vi "InternalResistance.vi"   [LabVIEW 2015]
uses:
  Formula Hybrid 2012 r1/Global Data.vi
  <vilib>/Platform/TimedLoop/XDataNode/XDataNode.xnode
  <vilib>/Platform/TimedLoop/XDataNode/nitl_modes.ctl
  <vilib>/Platform/TimedLoop/XDataNode/XDNodeRunTimeDep.lvlib
  <vilib>/Platform/TimedLoop/XDataNode/wakeup.ctl
  <vilib>/Platform/TimedLoop/XDataNode/timing_clust.ctl
types:
  T1 = typedef "XDNodeRunTimeDep.lvlib/timing_clust.ctl" = cluster{"Expected End [f-1]":u64, "Actual End [f-1]":u64, "Finished Late? [f-1]":bool, "Expected End [i-1]":u64, "Actual End [i-1]":u64, "Finished Late? [i-1]":bool, "Expected Start [i]":u64, "Actual Start [i]":u64, "Expected Start [f]":u64, "Actual Start [f]":u64, "Source Name":string, "Structure Name":string, "Period":i64, "Deadline":i64, "Offset":i64, "Start":i64, "Priority":i32, "Timeout":i32, "Mode":T2, "Wakeup Reason":T3, "Error":errorcluster, "Source Type":string, "Secondary Source Type":string, "Global End Time":u64, "Global Start Time":u64, "Frame Duration":u64, "Iteration Duration":u64, "Assigned CPU":i32, "I/O Scan Engine Mode":u32}
  T2 = typedef "XDNodeRunTimeDep.lvlib/nitl_modes.ctl" = enum32{"No Change", "Process missed periods, maintain original phase", "Discard missed periods, maintain original phase", "Process missed periods, ignore original phase", "Discard missed periods, ignore original phase"}
  T3 = typedef "XDNodeRunTimeDep.lvlib/wakeup.ctl" = enum32{"Normal", "Aborted", "Asynchronous wakeup", "Timing source error", "Timed loop error", "Timeout"}
  T4 = typedef "BMS Telemetry.ctl" = cluster{"bBMSIgnition":bool, "bBMSChargerMains":bool, "bBMSFastCharge":bool, "bBMSChargerEnabled":bool, "eBMSCarState":enum16{"Off", "On, Not Charging", "Charging", "Charging Finished", "Charging Error"}, "eBMSChargingState":enum16{"Disconnected", "Pre-charging", "Main Charging", "Balancing", "Charging Finished OK", "Charging Error"}, "tBMSChargeStage":u16, "eBMSLastChargeError":enum16{"No Error", "No Cell Communication", "No Cell Communication - Non CAN Charger", "Maximum charging stage duration expired", "Cell Communication Lost during Charge", "Cannot set balancing voltage", "Cell temps too high", "No Comms so can't determine temp", "# of Cells Mismatch", "Cells Overvoltage", "Cell Protection Event occured."}, "NBMSNumCells":u8, "bBMSUnderVProtection":bool, "bBMSOverVProtection":bool, "bBMSOverTProtection":bool, "bBMSLeakageProtection":bool, "bBMSNoCellCommsError":bool, "bBMSLowVReduction":bool, "bBMSHighTReduction":bool, "VCellMin":dbl, "VCellMax":dbl, "VCellMean":dbl, "VTotal":dbl, "TCellMin":dbl, "TCellMax":dbl, "TCellMean":dbl, "VCells":cluster{"[0]":dbl, "[1]":dbl, "[2]":dbl, "[3]":dbl, "[4]":dbl, "[5]":dbl, "[6]":dbl, "[7]":dbl, "[8]":dbl, "[9]":dbl, "[10]":dbl, "[11]":dbl, "[12]":dbl, "[13]":dbl, "[14]":dbl, "[15]":dbl, "[16]":dbl, "[16] 2":dbl, "[17]":dbl, "[18]":dbl, "[19]":dbl, "[20]":dbl, "[21]":dbl, "[22]":dbl, "[23]":dbl, "[24]":dbl, "[25]":dbl, "[26]":dbl, "[27]":dbl, "[28]":dbl, "[29]":dbl, "[30]":dbl, "[31]":dbl, "[32]":dbl, "[33]":dbl, "[33] 2":dbl, "[34]":dbl, "[35]":dbl, "[36]":dbl, "[37]":dbl, "[38]":dbl, "[39]":dbl, "[40]":dbl, "[41]":dbl, "[42]":dbl, "[43]":dbl, "[44]":dbl, "[45]":dbl, "[46]":dbl, "[47]":dbl, "[48]":dbl, "[49]":dbl, "[50]":dbl, "[50] 2":dbl, "[51]":dbl, "[52] 2":dbl, "[54]":dbl, "[53]":dbl, "[55]":dbl, "[56]":dbl, "[57]":dbl, "[58]":dbl, "[59]":dbl, "[60]":dbl, "[61]":dbl, "[62]":dbl, "[63]":dbl, "[64]":dbl, "[65]":dbl, "[66]":dbl, "[67]":dbl}, "TBMSCells":cluster{"[55]":dbl, "[56]":dbl, "[57]":dbl, "[58]":dbl, "[59]":dbl, "[60]":dbl, "[61]":dbl, "[62]":dbl, "[63]":dbl, "[64]":dbl, "[65]":dbl, "[66]":dbl, "[67]":dbl, "[68]":dbl, "[69]":dbl, "[70]":dbl, "[17]":dbl, "[38]":dbl, "[39]":dbl, "[40]":dbl, "[41]":dbl, "[42]":dbl, "[43]":dbl, "[44]":dbl, "[45]":dbl, "[46]":dbl, "[47]":dbl, "[48]":dbl, "[49]":dbl, "[50]":dbl, "[51]":dbl, "[52]":dbl, "[53]":dbl, "[54]":dbl, "[21]":dbl, "[22]":dbl, "[23]":dbl, "[24]":dbl, "[25]":dbl, "[26]":dbl, "[27]":dbl, "[28]":dbl, "[29]":dbl, "[30]":dbl, "[31]":dbl, "[32]":dbl, "[33]":dbl, "[34]":dbl, "[35]":dbl, "[36]":dbl, "[37]":dbl, "[0]":dbl, "[1]":dbl, "[2]":dbl, "[3]":dbl, "[4]":dbl, "[5]":dbl, "[6]":dbl, "[7]":dbl, "[8]":dbl, "[9]":dbl, "[10]":dbl, "[11]":dbl, "[12]":dbl, "[13]":dbl, "[14]":dbl, "[15]":dbl, "[16]":dbl}, "bChargerConnected":bool, "VChargerSetpoint":dbl, "IChargerSetpoint":dbl, "VChargerActual":dbl, "IChargerActual":dbl, "BCells":cluster{"[51]":dbl, "[52]":dbl, "[53]":dbl, "[54]":dbl, "[55]":dbl, "[56]":dbl, "[57]":dbl, "[58]":dbl, "[59]":dbl, "[60]":dbl, "[61]":dbl, "[62]":dbl, "[63]":dbl, "[64]":dbl, "[65]":dbl, "[66]":dbl, "[67]":dbl, "[34]":dbl, "[35]":dbl, "[36]":dbl, "[37]":dbl, "[38]":dbl, "[39]":dbl, "[40]":dbl, "[41]":dbl, "[42]":dbl, "[43]":dbl, "[44]":dbl, "[45]":dbl, "[46]":dbl, "[47]":dbl, "[48]":dbl, "[49]":dbl, "[50]":dbl, "[17]":dbl, "[18]":dbl, "[19]":dbl, "[20]":dbl, "[21]":dbl, "[22]":dbl, "[23]":dbl, "[24]":dbl, "[25]":dbl, "[26]":dbl, "[27]":dbl, "[28]":dbl, "[29]":dbl, "[30]":dbl, "[31]":dbl, "[32]":dbl, "[33]":dbl, "[0]":dbl, "[1]":dbl, "[2]":dbl, "[3]":dbl, "[4]":dbl, "[5]":dbl, "[6]":dbl, "[7]":dbl, "[8]":dbl, "[9]":dbl, "[10]":dbl, "[11]":dbl, "[12]":dbl, "[13]":dbl, "[14]":dbl, "[15]":dbl, "[16]":dbl}, "bNewVCellMinSample":bool, "Battery Temp":cluster{"[0]":dbl, "[1]":dbl, "[2]":dbl, "[3]":dbl, "[4]":dbl, "[5]":dbl, "[6]":dbl, "[7]":dbl, "[8]":dbl, "[9]":dbl, "[10]":dbl, "[11]":dbl, "[12]":dbl, "[13]":dbl, "[14]":dbl, "[15]":dbl, "[16]":dbl, "[17]":dbl, "[18]":dbl, "[19]":dbl, "[20]":dbl, "[21]":dbl, "[22]":dbl, "[23]":dbl, "[24]":dbl, "[25]":dbl, "[26]":dbl, "[27]":dbl, "[28]":dbl, "[29]":dbl, "[30]":dbl, "[31]":dbl, "[32]":dbl, "[33]":dbl, "[34]":dbl, "[35]":dbl, "[36]":dbl, "[37]":dbl, "[38]":dbl, "[39]":dbl, "[40]":dbl, "[41]":dbl, "[42]":dbl, "[43]":dbl, "[44]":dbl, "[45]":dbl, "[46]":dbl, "[47]":dbl, "[48]":dbl, "[49]":dbl, "[50]":dbl, "[51]":dbl, "[52]":dbl, "[53]":dbl, "[54]":dbl, "[55]":dbl, "[56]":dbl, "[57]":dbl, "[58]":dbl, "[59]":dbl, "[60]":dbl, "[61]":dbl, "[62]":dbl, "[63]":dbl, "[64]":dbl, "[65]":dbl, "[66]":dbl, "[67]":dbl, "[68]":dbl, "[69]":dbl, "[70]":dbl, "[71]":dbl, "[0] 2":dbl, "[1] 2":dbl, "[2] 2":dbl, "[3] 2":dbl, "[4] 2":dbl, "[5] 2":dbl, "[6] 2":dbl, "[7] 2":dbl, "[8] 2":dbl, "[9] 2":dbl, "[10] 2":dbl, "[11] 2":dbl, "[12] 2":dbl, "[13] 2":dbl, "[14] 2":dbl, "[15] 2":dbl, "[16] 2":dbl, "[17] 2":dbl, "[18] 2":dbl, "[19] 2":dbl, "[20] 2":dbl, "[21] 2":dbl, "[22] 2":dbl, "[23] 2":dbl, "[24] 2":dbl, "[25] 2":dbl, "[26] 2":dbl, "[27] 2":dbl, "[28] 2":dbl, "[29] 2":dbl, "[30] 2":dbl, "[31] 2":dbl, "[32] 2":dbl, "[33] 2":dbl, "[34] 2":dbl, "[35] 2":dbl, "[36] 2":dbl, "[37] 2":dbl, "[38] 2":dbl, "[39] 2":dbl, "[40] 2":dbl, "[41] 2":dbl, "[42] 2":dbl, "[43] 2":dbl, "[44] 2":dbl, "[45] 2":dbl, "[46] 2":dbl, "[47] 2":dbl, "[48] 2":dbl, "[49] 2":dbl, "[50] 2":dbl, "[51] 2":dbl, "[52] 3":dbl, "[53] 2":dbl, "[54] 2":dbl, "[55] 2":dbl, "[56] 2":dbl, "[57] 2":dbl, "[58] 2":dbl, "[59] 2":dbl, "[60] 2":dbl, "[61] 2":dbl, "[62] 2":dbl, "[63] 2":dbl, "[64] 2":dbl, "[65] 2":dbl, "[66] 2":dbl, "[67] 2":dbl, "[68]2":dbl, "[69]2":dbl, "[70]2":dbl, "[71]2":dbl, "[0] 3":dbl, "[1] 3":dbl, "[2] 3":dbl, "[3] 3":dbl, "[4] 3":dbl, "[5] 3":dbl, "[6] 3":dbl, "[7] 3":dbl, "[8] 3":dbl, "[9] 3":dbl, "[10] 3":dbl, "[11] 3":dbl, "[12] 3":dbl, "[13] 3":dbl, "[14] 3":dbl, "[15] 3":dbl, "[16] 3":dbl, "[17] 3":dbl, "[18] 3":dbl, "[19] 3":dbl, "[20] 3":dbl, "[21] 3":dbl, "[22] 3":dbl, "[23] 3":dbl, "[24] 3":dbl, "[25] 3":dbl, "[26] 3":dbl, "[27] 3":dbl, "[28] 3":dbl, "[29] 3":dbl, "[30] 3":dbl, "[31] 3":dbl, "[32] 3":dbl, "[33] 3":dbl, "[34] 3":dbl, "[35] 3":dbl, "[36] 3":dbl, "[37] 3":dbl, "[38] 3":dbl, "[39] 3":dbl, "[40] 3":dbl, "[41] 3":dbl, "[42] 3":dbl, "[43] 3":dbl, "[44] 3":dbl, "[45] 3":dbl, "[46] 3":dbl, "[47] 3":dbl, "[48] 3":dbl, "[49] 3":dbl, "[50] 3":dbl, "[51] 3":dbl, "[52] 4":dbl, "[53] 3":dbl, "[54] 3":dbl, "[55] 3":dbl, "[56] 3":dbl, "[57] 3":dbl, "[58] 3":dbl, "[59] 3":dbl, "[60] 3":dbl, "[61] 3":dbl, "[62] 3":dbl, "[63] 3":dbl, "[64] 3":dbl, "[65] 3":dbl, "[66] 3":dbl, "[67] 3":dbl, "[68]3":dbl, "[69]3":dbl, "[70]3":dbl, "[71]3":dbl, "[4] 4":dbl, "[5] 4":dbl, "[6] 4":dbl, "[7] 4":dbl, "[8] 4":dbl, "[9] 4":dbl, "[10] 4":dbl, "[11] 4":dbl, "[12] 4":dbl, "[13] 4":dbl, "[14] 4":dbl, "[15] 4":dbl, "[16] 4":dbl, "[17] 4":dbl, "[18] 4":dbl, "[19] 4":dbl, "[20] 4":dbl, "[21] 4":dbl, "[22] 4":dbl, "[23] 4":dbl, "[24] 4":dbl, "[25] 4":dbl, "[26] 4":dbl, "[27] 4":dbl, "[28] 4":dbl, "[29] 4":dbl, "[30] 4":dbl, "[31] 4":dbl, "[32] 4":dbl, "[33] 4":dbl, "[17] 9":dbl, "[0] 9":dbl, "[51] 8":dbl, "[34] 8":dbl, "[17] 8":dbl, "[0] 8":dbl, "[34] 4":dbl, "[35] 4":dbl, "[36] 4":dbl, "[37] 4":dbl, "[38] 4":dbl, "[39] 4":dbl, "[40] 4":dbl, "[41] 4":dbl, "[42] 4":dbl, "[43] 4":dbl, "[44] 4":dbl, "[45] 4":dbl, "[46] 4":dbl, "[47] 4":dbl, "[48] 4":dbl, "[49] 4":dbl, "[50] 4":dbl, "[34] 9":dbl, "[51] 4":dbl, "[52] 5":dbl, "[53] 4":dbl, "[54] 4":dbl, "[55] 4":dbl, "[56] 4":dbl, "[57] 4":dbl, "[58] 4":dbl, "[59] 4":dbl, "[60] 4":dbl, "[61] 4":dbl, "[62] 4":dbl, "[63] 4":dbl, "[64] 4":dbl, "[65] 4":dbl, "[66] 4":dbl, "[67] 4":dbl, "[51] 9":dbl}, "TBMSMax":dbl, "TBMSMin":dbl, "TBMSMean":dbl}
  T5 = typedef "FPGA Telemetry.ctl" = cluster{"CPU Load":cluster{"Total (%)":dbl, "Time Critical (%)":dbl, "Timed Structures (%)":dbl, "High (%)":dbl, "Above Normal (%)":dbl, "Normal (%)":dbl, "Background (%)":dbl, "Idle (%)":dbl, "ISR (%)":dbl}, "SVehicleStatus":cluster{"BMS Status":T6, "MC Status":T6, "Shutdown Status":T6, "sbRIO Status":T6, "Vehicle Status":T6, "Shutdown State":enum16{"NI.SC.Initial", "NI.SC.History", "NI.SC.ShallowHistory", "NI.SC.Terminal", "Coolant Pump Started/AIR's On", "AIRs On", "Precharge", "TSMS Off"}, "AIR Status":T9, "Remote Return to Pits":bool, "Reason for Shutdown":T10, "MC State Machine Status":enum16{"NI.SC.Initial", "NI.SC.History", "NI.SC.ShallowHistory", "NI.SC.Terminal", "Broadcast Diag", "Let Current Drop then Disable AIR's", "Enabled", "Disabled"}}, "iPhone HF Data":cluster{"gXiPhone":dbl, "gYiPhone":dbl, "gZiPhone":dbl, "nYawXiPhone":dbl, "nYawYiPhone":dbl, "nYawZiPhone":dbl}, "iPhone LF Data":cluster{"nLatiPhone":dbl, "nLongiPhone":dbl, "nGPSiPhone":dbl}, "stop":bool, "VSupplyOffset":fxp<+,12,4>, "VsbRIOSupply":fxp<+/-,25,6>, "bFPGALED":bool, "TSBRIO":fxp<+/-,33,17>, "rTPS2Unscaled":fxp<+/-,16,1>, "rTPS1Unscaled":fxp<+/-,16,1>, "bTPSConsistent":bool, "bTPSInRange":bool, "rThrottle":fxp<+/-,33,22>, "VTPS2":fxp<+/-,24,5>, "rTPS2":fxp<+/-,31,22>, "VTPS1":fxp<+/-,24,5>, "rTPS1":fxp<+/-,31,22>, "rTPS2Max":fxp<+,16,4>, "rTPS2Min":fxp<+,16,4>, "rTPS1Max":fxp<+,16,4>, "rTPS1Min":fxp<+,16,4>, "bCoolantPumpEnable":bool, "bRTDSEnable":bool, "bTSMSInStatus":bool, "bPosAIREnable":bool, "bBMSOK":bool, "bIMDOK":bool, "bBSPDOK":bool, "bSBRIOOK2":bool, "bSBRIOOK1":bool, "bTSMSOutStatus":bool, "eGreenDash":T11, "eYellowDash":T11, "eRedDash":T11, "bMotorControllerEnable":bool, "tCurrentLap":u32, "bNewLap":bool, "tLastLap":u32, "tLapMin":u32, "V5VSupply":fxp<+/-,24,5>, "bWheelRL":bool, "bWheelRR":bool, "bWheelFR":bool, "bWheelFL":bool, "VBrakePressureR":fxp<+/-,24,5>, "VBrakePressureF":fxp<+/-,24,5>, "bWheelRRStopped":bool, "bWheelRLStopped":bool, "bWheelFRStopped":bool, "bWheelFLStopped":bool, "tWheelRLPeriod":u32, "tWheelRRPeriod":u32, "tWheelFRPeriod":u32, "tWheelFLPeriod":u32, "bBrakeLight":bool, "VShockRR":fxp<+/-,24,5>, "VShockRL":fxp<+/-,24,5>, "VShockFR":fxp<+/-,24,5>, "VShockFL":fxp<+/-,24,5>, "IHighCurrent":fxp<+/-,24,15>, "ILowCurrent":fxp<+/-,24,15>, "pBrakeR":fxp<+,26,13>, "pBrakeF":fxp<+,26,13>, "bHighCurrentOK":bool, "bLowCurrentOK":bool, "bBrakeROK":bool, "bBrakeFOK":bool, "VSteerWheelMiddle":fxp<+/-,26,5>, "aSteerWheel":fxp<+/-,31,13>, "nWheelFL":fxp<+/-,32,16>, "nWheelFR":fxp<+/-,32,16>, "nWheelRL":fxp<+/-,32,16>, "nWheelRR":fxp<+/-,32,16>, "ADXL345 Output":T12, "Tire Diameter(m)":fxp<+,16,1>, "vWheelRR":fxp<+/-,32,18>, "vWheelRL":fxp<+/-,32,18>, "vWheelFR":fxp<+/-,32,18>, "vWheelFL":fxp<+/-,32,18>, "vWheelLowest":fxp<+/-,32,18>, "vWheelHighest":fxp<+/-,32,18>, "bAccel":bool, "vAxleF":fxp<+/-,33,19>, "vCar":fxp<+/-,33,19>, "sLap":fxp<+,32,12>, "rSlipRL":fxp<+/-,12,1>, "rSlipRR":fxp<+/-,12,1>, "rSlipFL":fxp<+/-,12,1>, "rSlipFR":fxp<+/-,12,1>, "NLap":u8, "tLapReference":u32, "tFastestLap":u32, "MTorqueRequest":dbl, "RS232 Error Out":cluster{"status":bool, "code":i32}}
  T6 = typedef "Subsystem Status.ctl" = cluster{"eStatusSeverity":T7, "NValue":sgl, "CMessage":T8, "bNotOK":bool}
  T7 = typedef "Subsystem Status Severity.ctl" = enum16{"Okay", "Short Warning", "Long Warning", "Return to Pits", "Error", "Danger"}
  T8 = typedef "Subsystem Status Message.ctl" = enum16{"ControllerTemperature", "MotorTemperature", "BatteryTemperature", "BatteryLowVoltage", "LVBattery", "sbRIOTemperature", "Precharge", "BSPD", "IMD", "RemoteReturnToPits", "EStopInterrupted", "NoCellComms", "MCOverSpeed", "MCOverCurrent", "MCOverVoltage", "MCInverterOverTemp", "MCDirectionCommand", "MCInverterTimeout", "MCDesatFault", "MCHWOverCurrent", "MCUnderVoltage", "MCCommandMessageLost", "MotorOverTemp", "MCModAOverTemp", "MCModBOverTemp", "MCModCOverTemp", "MCPCBOverTemp", "MCGateDrv1OverTemp", "MCDateDrv2OverTemp", "MCCurrentSensorFault", "MCResolverNotConnected", "ShutdownLatchTripped", "UnknownBMS", "RemoteEmergency"}
  T9 = typedef "AIR Status.ctl" = enum16{"Off", "Precharge", "On"}
  T10 = typedef "Reason for Shutdown.ctl" = enum16{"None", "BMS", "Shutdown", "sbRIO", "MC", "Remote"}
  T11 = typedef "Dash LED Status.ctl" = enum16{"Off", "Flashing", "On"}
  T12 = typedef "ADXL345 Output.ctl" = cluster{"X":fxp<+/-,14,4>, "Y":fxp<+/-,14,4>, "Z":fxp<+/-,14,4>}
  T13 = cluster{"[0]":dbl, "[1]":dbl, "[2]":dbl, "[3]":dbl, "[4]":dbl, "[5]":dbl, "[6]":dbl, "[7]":dbl, "[8]":dbl, "[9]":dbl, "[10]":dbl, "[11]":dbl, "[12]":dbl, "[13]":dbl, "[14]":dbl, "[15]":dbl, "[16]":dbl, "[16] 2":dbl, "[17]":dbl, "[18]":dbl, "[19]":dbl, "[20]":dbl, "[21]":dbl, "[22]":dbl, "[23]":dbl, "[24]":dbl, "[25]":dbl, "[26]":dbl, "[27]":dbl, "[28]":dbl, "[29]":dbl, "[30]":dbl, "[31]":dbl, "[32]":dbl, "[33]":dbl, "[33] 2":dbl, "[34]":dbl, "[35]":dbl, "[36]":dbl, "[37]":dbl, "[38]":dbl, "[39]":dbl, "[40]":dbl, "[41]":dbl, "[42]":dbl, "[43]":dbl, "[44]":dbl, "[45]":dbl, "[46]":dbl, "[47]":dbl, "[48]":dbl, "[49]":dbl, "[50]":dbl, "[50] 2":dbl, "[51]":dbl, "[52] 2":dbl, "[54]":dbl, "[53]":dbl, "[55]":dbl, "[56]":dbl, "[57]":dbl, "[58]":dbl, "[59]":dbl, "[60]":dbl, "[61]":dbl, "[62]":dbl, "[63]":dbl, "[64]":dbl, "[65]":dbl, "[66]":dbl, "[67]":dbl}
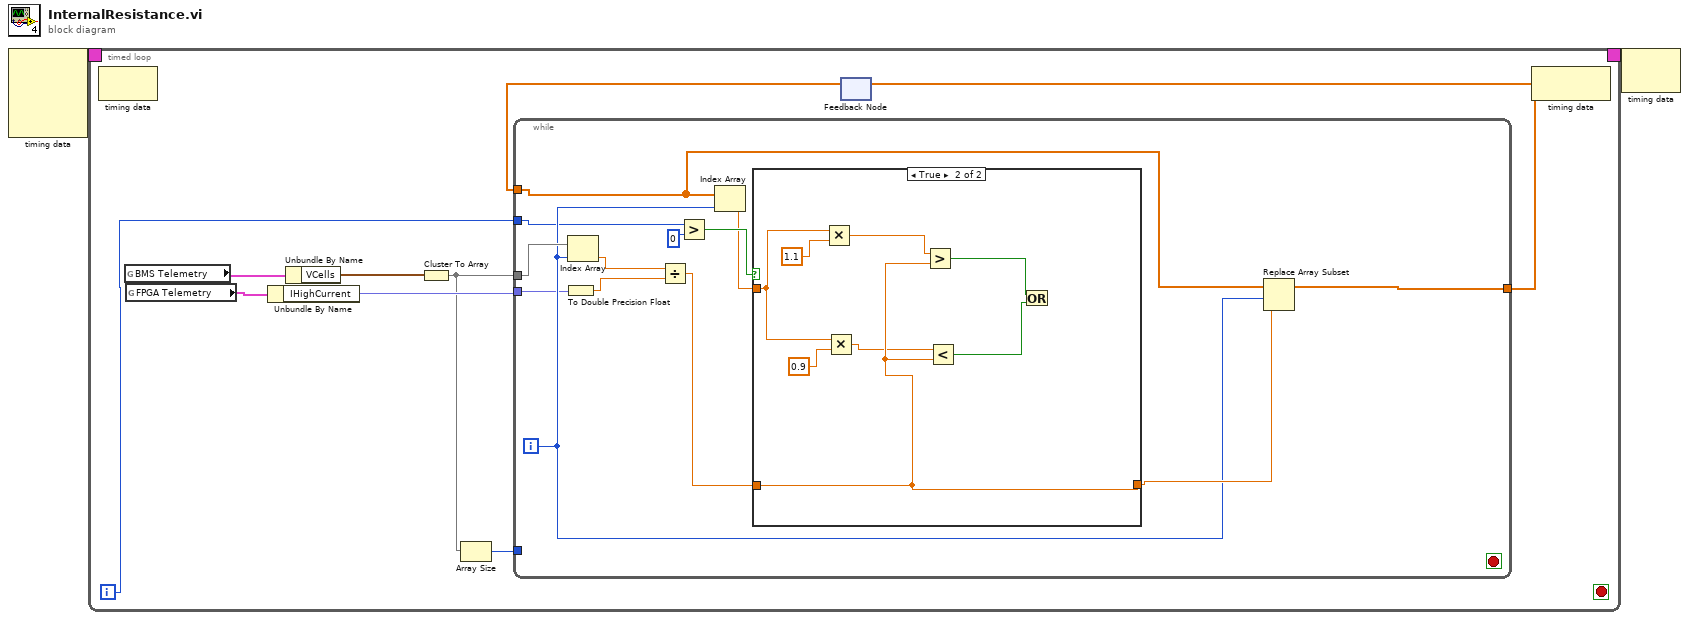
[diagram p0: block diagram]
diagram:
  n1 = node-c288() -> (w2:T1)  [unwired: 4 in]
  n2 = timed-loop {
    timing: w2 -> [_]
    timing-out: [_] -> w1
    i -> [w5]
    stop <- _ stop-if-true
    n3 = node-c288() -> ()  [unwired: 1 in, 1 out]
    n4 = global read "Global Data.vi" "BMS Telemetry"() -> (w11:T4)
    n5 = global read "Global Data.vi" "FPGA Telemetry"() -> (w7:T5)
    n6 = Unbundle By Name(w7) -> ("IHighCurrent"=w6:fxp<+/-,24,15>)
    n7 = Unbundle By Name(w11) -> ("VCells"=w10:T13)
    n8 = Cluster To Array(cluster=w10) -> (array=w4:dbl[])
    n9 = Array Size(array=w4) -> (size(s)=w3:i32)
    n10 = feedback #1() -> (w8:dbl[])  [unwired: 1 in]
    n11 = while {
      tunnel: w4 -> [w25]
      tunnel: w6 -> [w15]
      tunnel: [w17] -> w9
      tunnel: w8 -> [w16]
      tunnel: w5 -> [w13]
      tunnel: [w12] -> _
      tunnel: w3 -> [w12]
      i -> [w18]
      stop <- _ stop-if-true
      n12 = To Double Precision Float(number=w15) -> (double precision float=w14:dbl)
      n13 = Index Array(array=w25, index=w18) -> (element=w24:dbl)
      n14 = Divide(x=w24, y=w14) -> (x/y=w21:dbl)
      n15 = Greater?(x=w13, y=0) -> (0:w22:bool)
      n16 = Index Array(array=w16, index=w18) -> (element=w20:dbl)
      n17 = case shown="True" w22 {
        tunnel: w21 -> [w26 w31]
        tunnel: w20 -> [_ w32]
        tunnel: [w26 w31] -> w19
        frame False {
        }
        frame True {
          n18 = Multiply(x=w32, y=1.1) -> (x*y=w29:dbl)
          n19 = Multiply(x=w32, y=0.9) -> (x*y=w30:dbl)
          n20 = Greater?(x=w29, y=w31) -> (0:w34:bool)
          n21 = Less?(x=w30, y=w31) -> (x < y?=w33:bool)
          n22 = Or(x=w34, y=w33) -> ()  [unwired: 1 out]
        }
      }
      n23 = Replace Array Subset(array=w16, new element=w19, index=w18) -> (w17:dbl[])
    }
    n24 = feedback-in #1(w9) -> ()
    n25 = node-c288() -> ()  [unwired: 1 in, 1 out]
  }
  n26 = node-c288(w1) -> ()  [unwired: 1 out]
